vi "Z900_navX_Get_SystemInformation_BoardInformation.vi"(8 "error in (no error)":errorcluster, 11 "navX Device":T4={"Interface"={"Protocol"=enum."SERIAL", "Update Rate (4Hz-60Hz)"=4, "navX Open TypeDef"=variant}, "Notify Packet"=refnum, "Loop VI Refnum"=refnum} {"Interface"."Update Rate (4Hz-60Hz)" min=4 max=60 step=1}) -> (0 "error out":errorcluster, 2 "Board Information":T3 {"Board"."Hardware Revision" items=["navX-MXP"=33, "navX-Micro"=40]; "Omnimount Config" items=["DEFAULT", "X_UP", "X_DOWN", "Y_UP", "Y_DOWN", "Z_UP", "Z_DOWN"]}, 3 "navX Device":T4={"Interface"={"Protocol"=enum."SERIAL", "Update Rate (4Hz-60Hz)"=4, "navX Open TypeDef"=variant}, "Notify Packet"=refnum, "Loop VI Refnum"=refnum} {"Interface"."Update Rate (4Hz-60Hz)" min=4 max=60 step=1})   [LabVIEW 2014, in "navX Library v2.lvlib"]
uses:
  navX Library v2.lvlib
  TypeDefs/Z900_navX_DeviceTypeDef.ctl
  TypeDefs/Z900_navX_ProtocolTypeDef.ctl
  TypeDefs/Z900_navX_NotifyPacketTypeDef.ctl
  TypeDefs/Z900_navX_ActionTypeDef.ctl
  TypeDefs/Flags/Z900_navX_Flags_HardwareRevTypeDef.ctl
  TypeDefs/Flags/Z900_navX_Flags_OmnimountConfigTypeDef.ctl
  TypeDefs/Z900_navX_DeviceRegisters.ctl
  TypeDefs/Flags/Z900_navX_Flags_CapabilityTypeDef.ctl
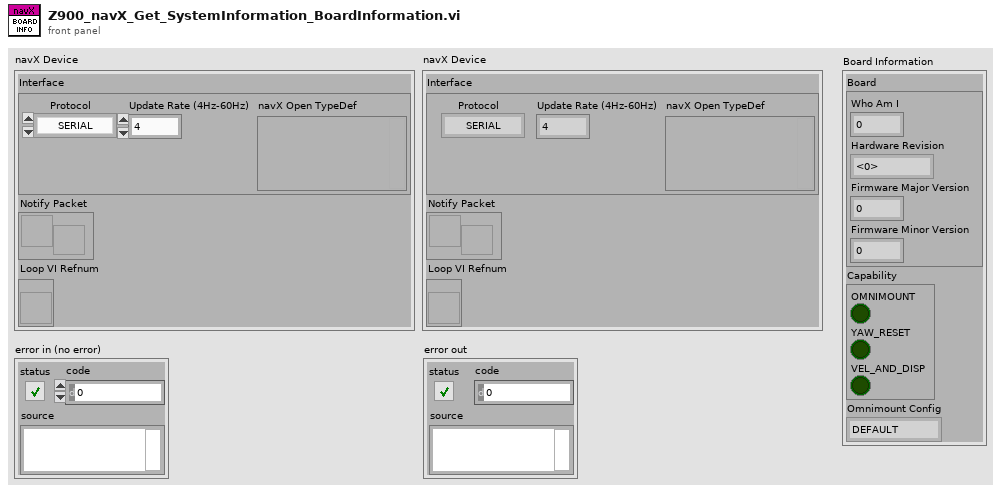
[diagram p1: front panel]
types:
  T1 = typedef "navX Library v2.lvlib/Z900_navX_Flags_HardwareRevTypeDef.ctl" = u8
  T2 = typedef "navX Library v2.lvlib/Z900_navX_Flags_OmnimountConfigTypeDef.ctl" = u8
  T3 = cluster{"Board":cluster{"Who Am I":u8, "Hardware Revision":T1, "Firmware Major Version":u8, "Firmware Minor Version":u8}, "Capability":cluster{"OMNIMOUNT":bool, "YAW_RESET":bool, "VEL_AND_DISP":bool}, "Omnimount Config":T2}
  T4 = typedef "navX Library v2.lvlib/Z900_navX_DeviceTypeDef.ctl" = cluster{"Interface":cluster{"Protocol":T5, "Update Rate (4Hz-60Hz)":u8, "navX Open TypeDef":variant}, "Notify Packet":refnum<notifier>, "Loop VI Refnum":refnum<vi>}
  T5 = typedef "navX Library v2.lvlib/Z900_navX_ProtocolTypeDef.ctl" = enum16{"SERIAL", "I2C", "SPI"}
  T6 = cluster{"Who Am I":u8, "Hardware Revision":T1, "Firmware Major Version":u8, "Firmware Minor Version":u8}
  T7 = cluster{"OMNIMOUNT":bool, "YAW_RESET":bool, "VEL_AND_DISP":bool}
  T8 = typedef "navX Library v2.lvlib/Z900_navX_DeviceRegisters.ctl" = u8
  T9 = typedef "navX Library v2.lvlib/Z900_navX_Flags_CapabilityTypeDef.ctl" = u16
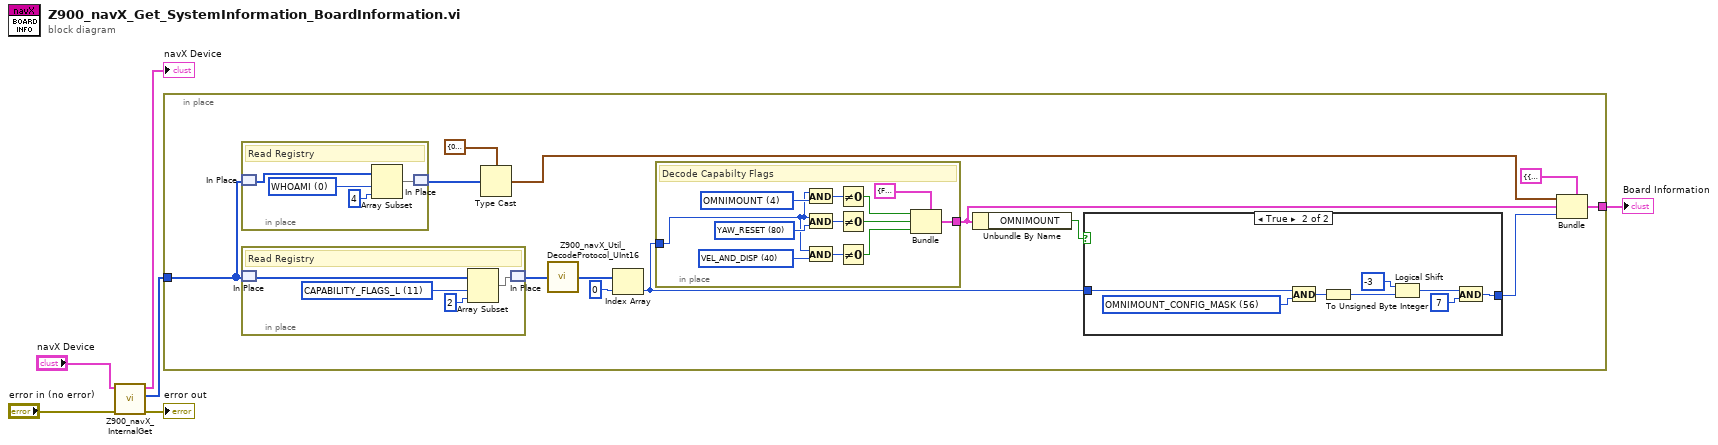
[diagram p0: block diagram]
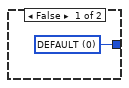
[diagram p2: hidden frame]
diagram:
  n1 = call "Z900_navX_InternalGet.vi"("error in (no error)"="error in (no error)", "navX Device"="navX Device") -> ("error out"=→"error out":errorcluster, "Local Registry"=w2:u8[], "navX Device"=→"navX Device":T4)  [unwired: 7 in]
  n2 = in-place {
    in-place-border: w2 -> [w15]
    in-place-border: [w9] -> w1
    n3 = in-place {
      w22 = T8 0 items=["WHOAMI"=0, "HW_REV"=1, "FW_VER_MAJOR"=2, "FW_VER_MINOR"=3, "UPDATE_RATE_HZ"=4, "ACCEL_FSR_G"=5, "GYRO_FSR_DPS"=6, "OP_STATUS"=8, "CAL_STATUS"=9, "SELFTEST_STATUS"=10, "CAPABILITY_FLAGS_L"=11, "CAPABILITY_FLAGS_H"=12, "SENSOR_STATUS"=16, "TIMESTAMP"=18, "YAW"=22, "ROLL"=24, "PITCH"=26, "HEADING"=28, "FUSED_HEADING"=30, "ALTITUDE_I"=32, "ALTITUDE_D"=34, "LINERA_ACC_X"=36, "LINERA_ACC_Y"=38, "LINERA_ACC_Z"=40, "QUAT_W"=42, "QUAT_X"=44, "QUAT_Y"=46, "QUAT_Z"=48, "MPU_TEMP_C"=50, "GYRO_X"=52, "GYRO_Y"=54, "GYRO_Z"=56, "ACC_X"=58, "ACC_Y"=60, "ACC_Z"=62, "MAG_X"=64, "MAG_Y"=66, "MAG_Z"=68, "PRESSURE_I"=70, "PRESSURE_D"=72, "PRESSURE_TEMP"=74, "YAW_OFFSET"=76, "QUAT_OFFSET_W"=78, "QUAT_OFFSET_X"=80, "QUAT_OFFSET_Y"=82, "QUAT_OFFSET_Z"=84, "INTEGRATION_CONTROL"=86, "VELOCITY_X"=88, "VELOCITY_Y"=92, "VELOCITY_Z"=96, "DISPLACMENT_X"=100, "DISPLACMENT_Y"=104, "DISPLACEMENT_Z"=108] ("Device Register")
      # "Read Registry"
      n4 = in-place-match #1(w15) -> (w20:u8[])
      n5 = Array Subset(array=w20, index=w22, length=4) -> (w21:u8[])
      n6 = in-place-match #1(w21) -> (w14:u8[])
    }
    n7 = in-place {
      w47 = T8 11 items=["WHOAMI"=0, "HW_REV"=1, "FW_VER_MAJOR"=2, "FW_VER_MINOR"=3, "UPDATE_RATE_HZ"=4, "ACCEL_FSR_G"=5, "GYRO_FSR_DPS"=6, "OP_STATUS"=8, "CAL_STATUS"=9, "SELFTEST_STATUS"=10, "CAPABILITY_FLAGS_L"=11, "CAPABILITY_FLAGS_H"=12, "SENSOR_STATUS"=16, "TIMESTAMP"=18, "YAW"=22, "ROLL"=24, "PITCH"=26, "HEADING"=28, "FUSED_HEADING"=30, "ALTITUDE_I"=32, "ALTITUDE_D"=34, "LINERA_ACC_X"=36, "LINERA_ACC_Y"=38, "LINERA_ACC_Z"=40, "QUAT_W"=42, "QUAT_X"=44, "QUAT_Y"=46, "QUAT_Z"=48, "MPU_TEMP_C"=50, "GYRO_X"=52, "GYRO_Y"=54, "GYRO_Z"=56, "ACC_X"=58, "ACC_Y"=60, "ACC_Z"=62, "MAG_X"=64, "MAG_Y"=66, "MAG_Z"=68, "PRESSURE_I"=70, "PRESSURE_D"=72, "PRESSURE_TEMP"=74, "YAW_OFFSET"=76, "QUAT_OFFSET_W"=78, "QUAT_OFFSET_X"=80, "QUAT_OFFSET_Y"=82, "QUAT_OFFSET_Z"=84, "INTEGRATION_CONTROL"=86, "VELOCITY_X"=88, "VELOCITY_Y"=92, "VELOCITY_Z"=96, "DISPLACMENT_X"=100, "DISPLACMENT_Y"=104, "DISPLACEMENT_Z"=108] ("Device Register")
      # "Read Registry"
      n8 = in-place-match #2(w15) -> (w45:u8[])
      n9 = Array Subset(array=w45, index=w47, length=2) -> (w46:u8[])
      n10 = in-place-match #2(w46) -> (w19:u8[])
    }
    n11 = Type Cast(type=T6 {"Who Am I"=0, "Hardware Revision"=33, "Firmware Major Version"=0, "Firmware Minor Version"=0}, x=w14) -> (*(type *) &x=w10:T6)
    n12 = call "Z900_navX_Util_DecodeProtocol_UInt16.vi"("Little Endian"=w19) -> ("UInt16"=w18:u16[])
    n13 = Index Array(array=w18, index=0) -> (element=w17:u16)
    n14 = in-place {
      in-place-border: w17 -> [w35]
      in-place-border: [w33] -> w11
      w38 = T9 40 items=["OMNIMOUNT"=4, "OMNIMOUNT_CONFIG_MASK"=38, "VEL_AND_DISP"=40, "YAW_RESET"=80] ("Capability Flag")
      w39 = T9 80 items=["OMNIMOUNT"=4, "OMNIMOUNT_CONFIG_MASK"=38, "VEL_AND_DISP"=40, "YAW_RESET"=80] ("Capability Flag")
      w44 = T9 4 items=["OMNIMOUNT"=4, "OMNIMOUNT_CONFIG_MASK"=38, "VEL_AND_DISP"=40, "YAW_RESET"=80] ("Capability Flag")
      # "Decode Capabilty Flags"
      n15 = And(x=w35, y=w44) -> (x .and. y?=w43:T9)
      n16 = And(x=w35, y=w39) -> (x .and. y?=w40:T9)
      n17 = And(x=w35, y=w38) -> (x .and. y?=w37:T9)
      n18 = Not Equal To 0?(x=w43) -> (x != 0?=w41:bool)
      n19 = Not Equal To 0?(x=w40) -> (x != 0?=w36:bool)
      n20 = Not Equal To 0?(x=w37) -> (x != 0?=w34:bool)
      n21 = Bundle(cluster=T7 {"OMNIMOUNT"=FALSE, "YAW_RESET"=FALSE, "VEL_AND_DISP"=FALSE}, "OMNIMOUNT"=w41, "YAW_RESET"=w36, "VEL_AND_DISP"=w34) -> (w33:T7)
    }
    n22 = Unbundle By Name(w11) -> ("OMNIMOUNT"=w16:bool)
    n23 = case shown="True" w16 {
      tunnel: [w24 w26] -> w7
      tunnel: w17 -> [_ w32]
      frame False {
        w24 = u8 0 items=["DEFAULT", "X_UP", "X_DOWN", "Y_UP", "Y_DOWN", "Z_UP", "Z_DOWN"] ("OMNIMOUNT_CONFIG")
      }
      frame True {
        w31 = T9 56 items=["OMNIMOUNT"=4, "OMNIMOUNT_CONFIG_MASK"=56, "VEL_AND_DISP"=64, "YAW_RESET"=128] ("Capability Flag")
        n24 = And(x=w32, y=w31) -> (x .and. y?=w30:T9)
        n25 = To Unsigned Byte Integer(number=w30) -> (unsigned 8bit integer=w25:u8)
        n26 = Logical Shift(y=-3, x=w25) -> (x << y=w28:u8)
        n27 = And(x=w28, y=7) -> (x .and. y?=w26:i32)
      }
    }
    n28 = Bundle(cluster=T3 {"Board"={"Who Am I"=0, "Hardware Revision"=33, "Firmware Major Version"=0, "Firmware Minor Version"=0}, "Capability"={"OMNIMOUNT"=FALSE, "YAW_RESET"=FALSE, "VEL_AND_DISP"=FALSE}, "Omnimount Config"=0}, "Board"=w10, "Capability"=w11, "Omnimount Config"=w7) -> (w9:T3)
  }
  "Board Information" <- w1
